vi "Do.vi"(8 "error in (no error)":errorcluster, 10 "FormulaG API":refnum<class "FormulaG API.lvclass">, 11 "UI Options Cmd in":refnum<class "UI Options Cmd.lvclass">) -> (0 "error out":errorcluster, 3 "UI Options Cmd out":refnum<class "UI Options Cmd.lvclass">)   [LabVIEW 2020, in "FormulaG.lvlib" / "UI Options Cmd.lvclass"]
uses:
  UI Options Cmd.lvclass
  FormulaG API/FormulaG API.lvclass
  UI Options Cmd.lvclass/UI Options Cmd.ctl
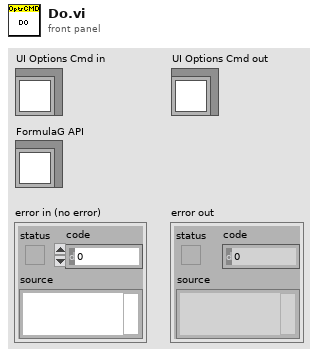
[diagram p1: front panel]
types:
  T1 = typedef "FormulaG-Common.lvlib/UI Options.ctl" = cluster{"Range Visible":bool}
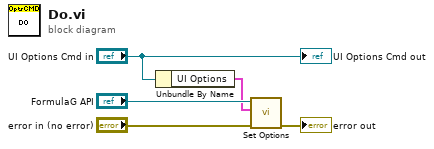
[diagram p0: block diagram]
diagram:
  n1 = Unbundle By Name("UI Options Cmd in") -> ("UI Options"=w1:T1)
  n2 = call "Set Options.vi"("error in (no error)"="error in (no error)", "UI Options"=w1, "FormulaG API in"="FormulaG API") -> ("error out"=→"error out":errorcluster)  [unwired: 7 in, 1 out]
  "UI Options Cmd out" <- "UI Options Cmd in"
